vi "new.vi"(8 "error in (no error)":errorcluster, 9 "guid (\"\": generate new)":string, 10 "label (\"\")":string, 11 "Node in":refnum<class "Node.lvclass">) -> (0 "error out":errorcluster, 3 "Node out":refnum<class "Node.lvclass">)   [LabVIEW 2020, in "graph.lvlib" / "Node.lvclass"]
uses:
  Node.lvclass
  Node.lvclass/Node.ctl
  ID/ID.lvclass
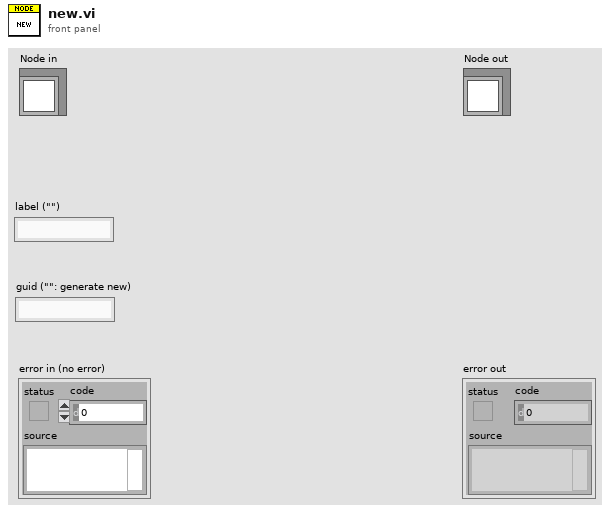
[diagram p1: front panel]
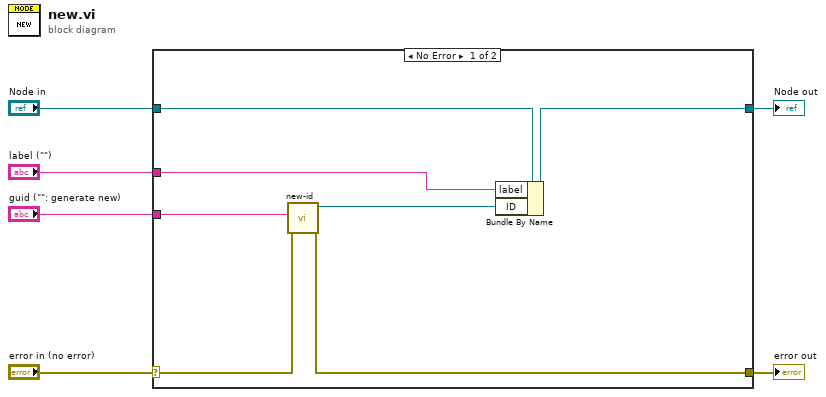
[diagram p0: block diagram]
diagram:
  n1 = case shown="No Error" "error in (no error)" {
    selector: "error in (no error)" -> [w10 w15]
    tunnel: [w9 w15] -> w5
    tunnel: [w12 w14] -> w3
    tunnel: "Node in" -> [w13 w14]
    tunnel: "guid (\"\": generate new)" -> [w8 _]
    tunnel: "label (\"\")" -> [w7 _]
    frame No Error {
      n2 = call "new-id.vi"("error in (no error)"=w10, "id-string (\"\": generate new id)"=w8) -> ("error out"=w9:errorcluster, "ID out"=w11:refnum<class "ID.lvclass">)  [unwired: 8 in]
      n3 = Bundle By Name(cluster=w13, "label"=w7, "ID"=w11) -> (w12:refnum<class "Node.lvclass">)
    }
    frame Error {
    }
  }
  "error out" <- w5
  "Node out" <- w3
